vi "Ophir_calibration.vi"(10 "Адрес Ophir":refnum<visa-resource-name>="USB0::0x0BD3::0x0777::NI-VISA-10005::RAW", 11 "Путь к калибровке":path=path "D:/#mech/LVPROG/1991_Маэстро/Калибровка/Proj/Осциллограммы") -> ()   [LabVIEW 2013]
uses:
  <vilib>/Analysis/baseanly.llb/Mean (DBL).vi
  <vilib>/Utility/file.llb/Write To Spreadsheet File (DBL).vi
  <vilib>/Analysis/NI_AALBase.lvlib
panel:
  in  "X6 (N10)":dbl[][](array[numeric])=[[0.1, 2.0], [0.5, 2.0], [1.0, 2.0], [3.0, 2.0], [5.0, 2.0], [10.0, 2.0], [15.0, 2.0], [20.0, 2.0], [25.0, 2.0], [30.0, 2.0], [35.0, 2.0], [40.0, 2.0], [45.0, 20.0], [50.0, 20.0], [55.0, 20.0], [60.0, 20.0], [65.0, 20.0], [70.0, 20.0], [75.0, 20.0], [80.0, 20.0], [85.0, 20.0], [90.0, 20.0], [95.0, 20.0], [100.0, 20.0]] format="%0.3f"
  in  "Количество прострелов в импульсе":i32=40
  out "Минут":dbl=17.886183333333335
  in  "Boolean":bool=TRUE
  out "Предел":string="3"
  out "mean":dbl=2.91575 format="%0.2f"
  out "number 2":dbl=3.22e-06
  in  "number":i32
  out "Результат":string="*\n\n"
  in  "Телескоп":enum16{"X6", "X3", "X2", "X1"}(ring)
  in  "X1":dbl[][](array[numeric])=[[0.1, 20.0], [0.5, 200.0], [1.0, 200.0], [3.0, 2000.0], [5.0, 2000.0], [10.0, 2000.0], [15.0, 10000.0], [20.0, 10000.0], [25.0, 10000.0], [30.0, 10000.0], [35.0, 10000.0], [40.0, 10000.0], [45.0, 10000.0], [50.0, 10000.0], [55.0, 10000.0], [60.0, 10000.0], [65.0, 10000.0], [70.0, 10000.0], [75.0, 10000.0], [80.0, 10000.0], [85.0, 10000.0], [90.0, 10000.0], [95.0, 10000.0], [100.0, 10000.0]] format="%0.3f"
  in  "X2":dbl[][](array[numeric])=[[0.1, 20.0], [0.5, 200.0], [1.0, 200.0], [3.0, 200.0], [5.0, 2000.0], [10.0, 2000.0], [15.0, 2000.0], [20.0, 2000.0], [25.0, 2000.0], [30.0, 2000.0], [35.0, 2000.0], [40.0, 2000.0], [45.0, 10000.0], [50.0, 10000.0], [55.0, 10000.0], [60.0, 10000.0], [65.0, 10000.0], [70.0, 10000.0], [75.0, 10000.0], [80.0, 10000.0], [85.0, 10000.0], [90.0, 10000.0], [95.0, 10000.0], [100.0, 10000.0]] format="%0.3f"
  in  "X3":dbl[][](array[numeric])=[[0.1, 20.0], [0.5, 20.0], [1.0, 200.0], [3.0, 200.0], [5.0, 200.0], [10.0, 2000.0], [15.0, 2000.0], [20.0, 2000.0], [25.0, 2000.0], [30.0, 2000.0], [35.0, 2000.0], [40.0, 2000.0], [45.0, 2000.0], [50.0, 2000.0], [55.0, 2000.0], [60.0, 2000.0], [65.0, 2000.0], [70.0, 2000.0], [75.0, 2000.0], [80.0, 2000.0], [85.0, 2000.0], [90.0, 2000.0], [95.0, 2000.0], [100.0, 2000.0]] format="%0.3f"
  in  "X6":dbl[][](array[numeric])=[[0.1, 2.0], [0.5, 20.0], [1.0, 20.0], [3.0, 20.0], [5.0, 200.0], [10.0, 200.0], [15.0, 200.0], [20.0, 200.0], [25.0, 200.0], [30.0, 200.0], [35.0, 200.0], [40.0, 200.0], [45.0, 200.0], [50.0, 200.0], [55.0, 200.0], [60.0, 200.0], [65.0, 200.0], [70.0, 2000.0], [75.0, 2000.0], [80.0, 2000.0], [85.0, 2000.0], [90.0, 2000.0], [95.0, 2000.0], [100.0, 2000.0]] format="%0.3f"
  in  "USB Channel number (default 0)":dbl
  out "XY Graph":cluster{dbl[], dbl[]}(graph)={[45.0, 46.0, 47.0, 48.0, 49.0, 50.0, 51.0, 52.0, 53.0, 54.0, 55.0, 56.0, 57.0, 58.0, 59.0, 60.0, 61.0, 62.0, 63.0, 64.0, 65.0, 66.0, 67.0, 68.0, 69.0, 70.0, 71.0, 72.0, 73.0, 74.0, 75.0, 76.0, 77.0, 78.0, 79.0], [5.82625, 5.09275, 5.42575, 5.7905, 1.9792500000000002, 3.1294999999999997, 2.85025, 2.0719999999999996, 1.9745, 2.1955, 1.99275, 2.2165, 2.0700000000000003, 2.3114999999999997, 2.2840000000000003, 2.29225, 2.153, 2.2262500000000003, 2.49075, 2.4105, 2.2475, 2.3665000000000003, 2.592, 2.55425, 2.43575, 2.7362499999999996, 2.6025, 2.5602500000000004, 2.5745, 2.8725, 2.713, 2.661, 2.85275, 2.81675, 2.91575]}
  out "Текущий процент, %":dbl=79.0
  out "Шаг, %":dbl=1.0
  in  "Диапазон/Точки":bool=TRUE
  in  "Точки":dbl[](array[numeric])
  in  "Максимальный процент, %":dbl=80.0
  in  "Минимальный процент, %":dbl=45.0
  in  "Количество точек":u32=35
  in  "But_Автопрострел":bool=TRUE
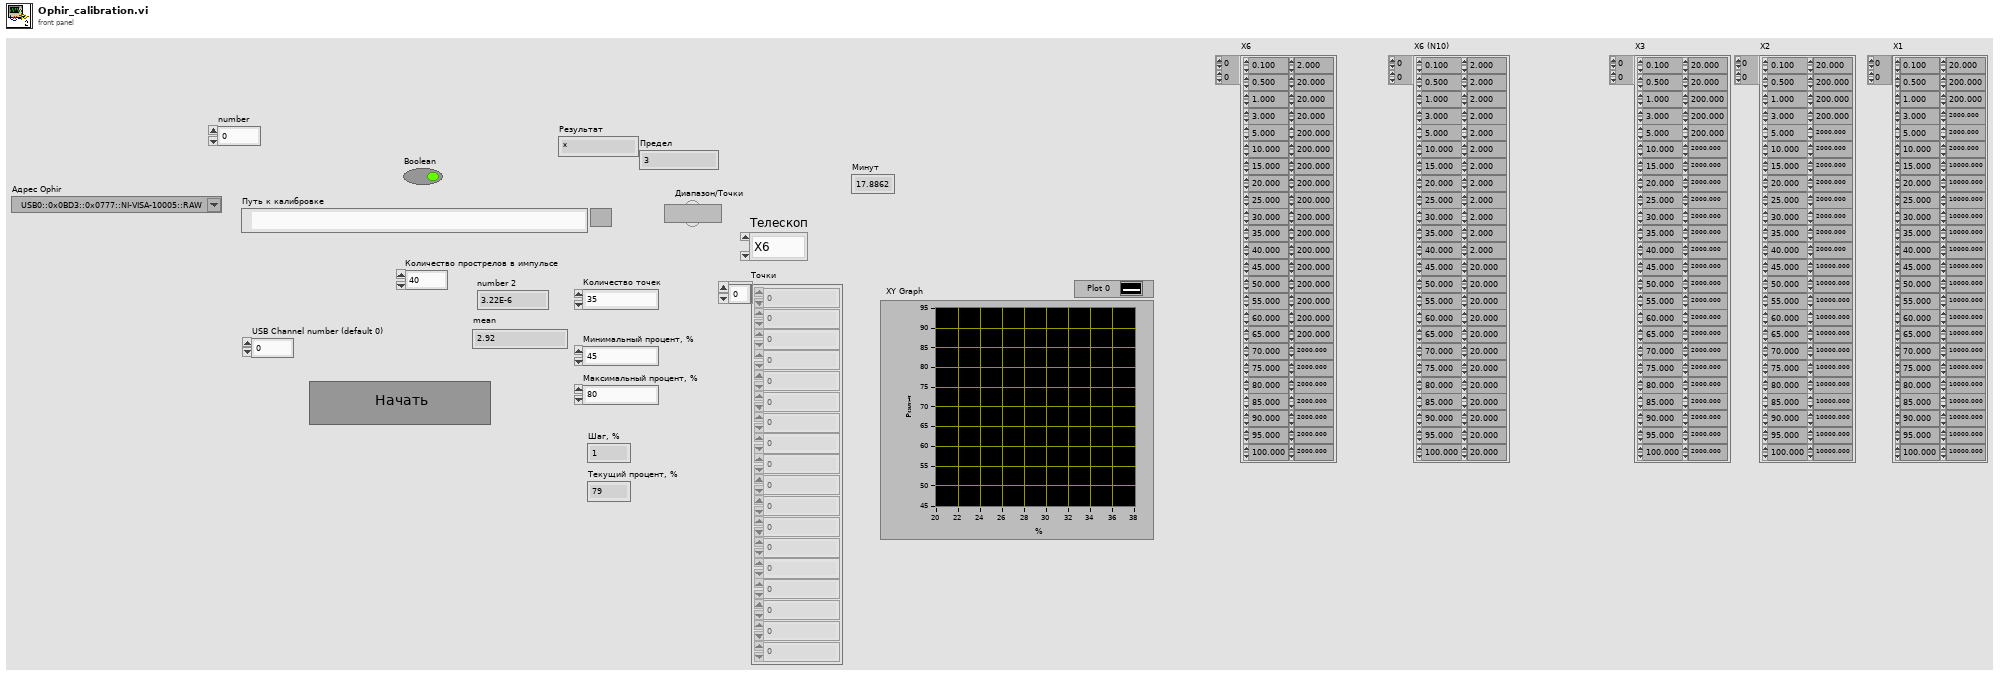
[diagram p1: front panel]
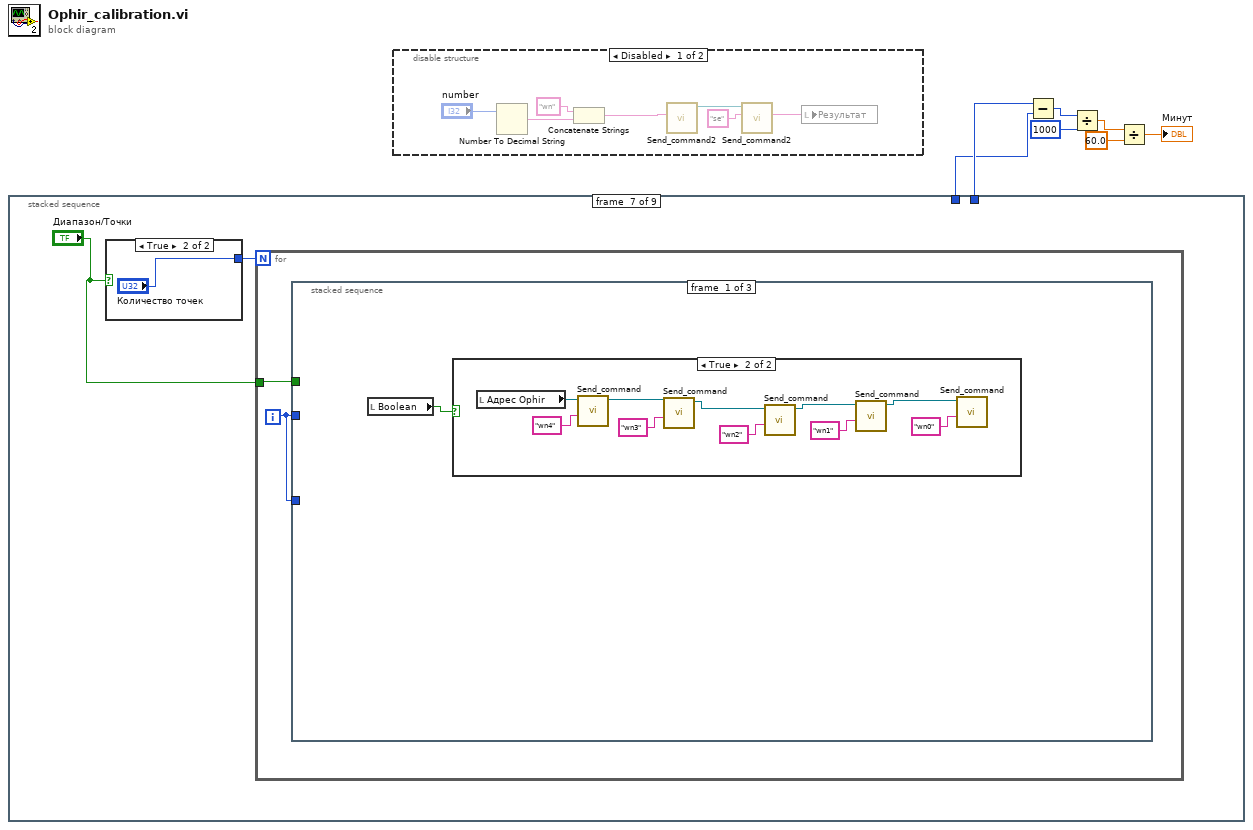
[diagram p0: block diagram]
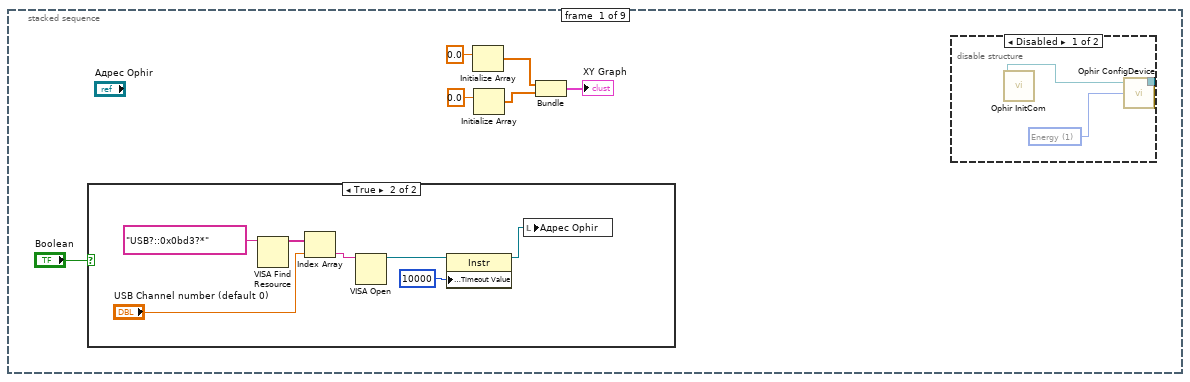
[diagram p3: hidden frame]
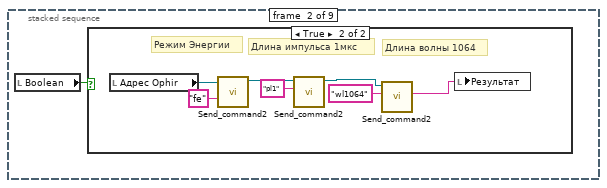
[diagram p6: hidden frame]
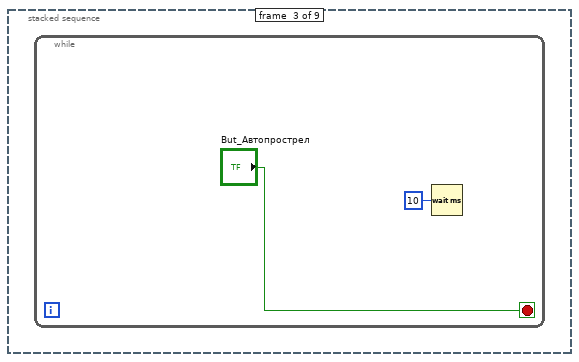
[diagram p8: hidden frame]
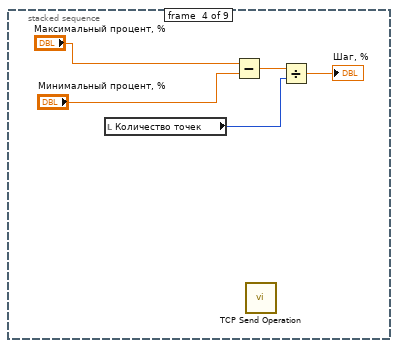
[diagram p9: hidden frame]
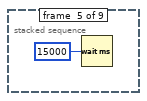
[diagram p10: hidden frame]
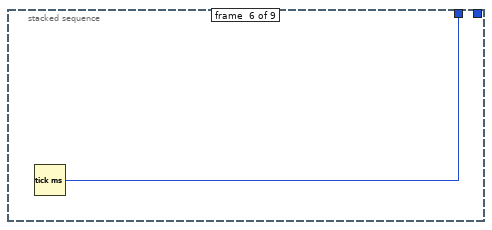
[diagram p11: hidden frame]
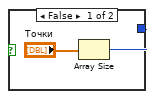
[diagram p12: hidden frame]
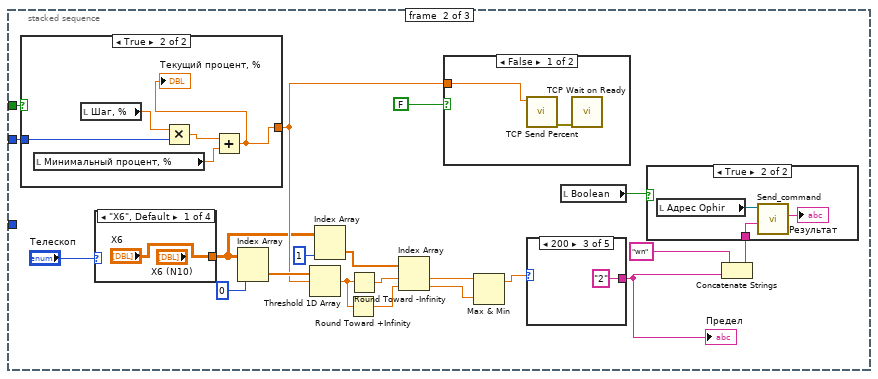
[diagram p14: hidden frame]
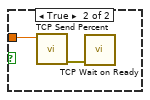
[diagram p16: hidden frame]
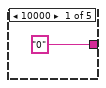
[diagram p17: hidden frame]
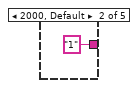
[diagram p18: hidden frame]
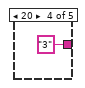
[diagram p19: hidden frame]
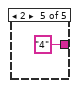
[diagram p20: hidden frame]
diagram:
  n1 = stacked-sequence {
    tunnel: [_ _ _ _ _ w40 _ _ _] -> w6
    tunnel: [_ _ _ _ _ _ _ w134 _] -> w7
    frame #0 {
      n2 = case shown="True" "Boolean" {
        frame False {
        }
        frame True {
          n3 = VISA Find Resource(11:"USB?::0x0bd3?*" ("USB0::0x0BD3")) -> (3:w16:string[])  [unwired: 1 in, 3 out]
          n4 = Index Array(array=w16, index="USB Channel number (default 0)") -> (element=w19:string)
          n5 = VISA Open(VISA resource name=w19) -> (VISA resource name=w20:refnum<visa-resource-name>)  [unwired: 1 in, 4 out]
          n6 = property class="Instr"(reference=w20, "General Settings:Timeout Value"=u32 10000) -> (reference out=w14:refnum<visa-resource-name>)  [unwired: 1 in, 1 out]
          n7 = local write "Адрес Ophir"(w14) -> ()
        }
      }
      n8 = Initialize Array(0.0 ("element")) -> (w11:dbl[])  [unwired: 1 in]
      n9 = Initialize Array(0.0 ("element")) -> (w10:dbl[])  [unwired: 1 in]
      n10 = Bundle(w11, w10) -> (→"XY Graph":cluster{dbl[], dbl[]})  [unwired: 1 in]
      n11 = disable-structure shown="Disabled" {
        disable-tunnel: [w21 _] -> _
        frame Disabled {
          w22 = u16 1 items=["Power", "Energy", "Frequency"] ("Measure Choice (0:Power)")
          n12 = call "Ophir InitCom.vi"() -> ("Visa Session"=w23:refnum<visa-resource-name>)  [unwired: 6 in, 2 out]
          n13 = call "Ophir ConfigDevice.vi"("Visa Session"=w23, "Measure Choice (0:Power)"=w22) -> ("dup Visa Session"=w21:refnum<visa-resource-name>)  [unwired: 1 in, 3 out]
        }
        frame Enabled {
        }
      }
    }
    frame #1 {
      n14 = local read "Boolean"() -> (w24:bool)
      n15 = case shown="True" w24 {
        frame False {
        }
        frame True {
          # "Длина волны 1064"
          # "Длина импульса 1мкс"
          # "Режим Энергии"
          n16 = local read "Адрес Ophir"() -> (w31:refnum<visa-resource-name>)
          n17 = call "Send_command2.vi"("String"="fe", "VISA Refnum in"=w31) -> ("VISA Refnum out"=w29:refnum<visa-resource-name>)  [unwired: 8 in, 1 out]
          n18 = call "Send_command2.vi"("String"="pl1", "VISA Refnum in"=w29) -> ("VISA Refnum out"=w26:refnum<visa-resource-name>)  [unwired: 8 in, 1 out]
          n19 = call "Send_command2.vi"("String"="wl1064", "VISA Refnum in"=w26) -> ("string"=w25:string)  [unwired: 8 in, 1 out]
          n20 = local write "Результат"(w25) -> ()
        }
      }
    }
    frame #2 {
      n21 = while {
        stop <- "But_Автопрострел" stop-if-true
        n22 = Wait (ms)(milliseconds to wait=u32 10) -> ()  [unwired: 1 out]
      }
    }
    frame #3 {
      n23 = local read "Количество точек"() -> (w37:u32)
      n24 = Subtract(x="Максимальный процент, %", y="Минимальный процент, %") -> (x-y=w36:dbl)
      n25 = call "TCP Send Operation.vi"() -> ()  [unwired: 11 in, 1 out]
      n26 = Divide(x=w36, y=w37) -> (x/y=→"Шаг, %":dbl)
    }
    frame #4 {
      n27 = Wait (ms)(milliseconds to wait=u32 15000) -> ()  [unwired: 1 out]
    }
    frame #5 {
      n28 = Tick Count (ms)() -> (millisecond timer value=w40:u32)
    }
    frame #6 {
      n29 = case shown="True" "Диапазон/Точки" {
        tunnel: [w43 "Количество точек"] -> w42
        frame False {
          n30 = Array Size(array="Точки") -> (size(s)=w43:i32)
        }
        frame True {
        }
      }
      n31 = for {
        N: w42 -> [_]
        tunnel: "Диапазон/Точки" -> [w47]
        i -> [w46]
        n32 = stacked-sequence {
          tunnel: w47 -> [_ w78 _]
          tunnel: w46 -> [_ w77 _]
          tunnel: w46 -> [_ _ w107]
          frame #0 {
            n33 = local read "Boolean"() -> (w48:bool)
            n34 = case shown="True" w48 {
              frame False {
              }
              frame True {
                n35 = local read "Адрес Ophir"() -> (w53:refnum<visa-resource-name>)
                n36 = call "Send_command.vi"("Команда"="wn4", "Адрес"=w53) -> ("Адрес 2"=w52:refnum<visa-resource-name>)  [unwired: 8 in, 1 out]
                n37 = call "Send_command.vi"("Команда"="wn3", "Адрес"=w52) -> ("Адрес 2"=w51:refnum<visa-resource-name>)  [unwired: 8 in, 1 out]
                n38 = call "Send_command.vi"("Команда"="wn2", "Адрес"=w51) -> ("Адрес 2"=w50:refnum<visa-resource-name>)  [unwired: 8 in, 1 out]
                n39 = call "Send_command.vi"("Команда"="wn1", "Адрес"=w50) -> ("Адрес 2"=w49:refnum<visa-resource-name>)  [unwired: 8 in, 1 out]
                n40 = call "Send_command.vi"("Команда"="wn0", "Адрес"=w49) -> ()  [unwired: 8 in, 2 out]
              }
            }
          }
          frame #1 {
            n41 = case shown="True" w78 {
              tunnel: w77 -> [w96 w100]
              tunnel: [w95 w98] -> w73
              frame False {
                n42 = local read "Точки"() -> (w97:dbl[])
                n43 = Index Array(array=w97, index=w96) -> (element=w95:dbl)
              }
              frame True {
                n44 = local read "Минимальный процент, %"() -> (w102:dbl)
                n45 = local read "Шаг, %"() -> (w101:dbl)
                n46 = Multiply(x=w101, y=w100) -> (x*y=w99:dbl)
                n47 = Add(x=w99, y=w102) -> (x+y=w98:dbl)
                "Текущий процент, %" <- w98
              }
            }
            n48 = case shown="\"X6\", Default" "Телескоп" {
              tunnel: ["X6" "X3" "X2" "X1"] -> w72
              frame "X6", Default {
              }
              frame "X3" {
              }
              frame "X2" {
              }
              frame "X1" {
              }
            }
            n49 = Index Array(array=w72, index (col)=0 ("disabled index (col)")) -> (element=w74:dbl[])  [unwired: 1 in]
            n50 = Threshold 1D Array(2:w73, 3:w74) -> (0:w68:dbl)  [unwired: 1 in]
            n51 = Index Array(array=w72, index (col)=1 ("disabled index (col)")) -> (element=w70:dbl[])  [unwired: 1 in]
            n52 = Round Toward +Infinity(x=w68) -> (ceil(x): smallest int >= x=w67:dbl)
            n53 = Round Toward -Infinity(1:w68) -> (0:w69:dbl)
            n54 = Index Array(array=w70, index #1=w69, index #2=w67) -> (element #1=w66:dbl, element #2=w65:dbl)
            n55 = case shown="False" FALSE {
              tunnel: w73 -> [w83 w84]
              frame False {
                n56 = call "TCP Send Percent.vi"("Percent"=w83) -> ("error out"=w82:errorcluster)  [unwired: 10 in]
                n57 = call "TCP Wait on Ready.vi"("error in"=w82) -> ()  [unwired: 9 in, 1 out]
              }
              frame True {
                n58 = call "TCP Send Percent.vi"("Percent"=w84) -> ("error out"=w85:errorcluster)  [unwired: 10 in]
                n59 = call "TCP Wait on Ready.vi"("error in"=w85) -> ()  [unwired: 9 in, 1 out]
              }
            }
            n60 = Max & Min(x=w66, y=w65) -> (max(x,y)=w64:dbl)  [unwired: 1 out]
            n61 = case shown="200" w64 {
              tunnel: ["0" "1" "2" "3" "4"] -> w62
              frame 10000 {
              }
              frame 2000, Default {
              }
              frame 200 {
              }
              frame 20 {
              }
              frame 2 {
              }
            }
            "Предел" <- w62
            n62 = local read "Boolean"() -> (w59:bool)
            n63 = Concatenate Strings("wn", w62) -> (w61:string)
            n64 = case shown="True" w59 {
              tunnel: w61 -> [_ w81]
              frame False {
              }
              frame True {
                n65 = local read "Адрес Ophir"() -> (w80:refnum<visa-resource-name>)
                n66 = call "Send_command.vi"("Команда"=w81, "Адрес"=w80) -> ("Результат"=→"Результат":string)  [unwired: 8 in, 1 out]
              }
            }
          }
          frame #2 {
            n67 = local read "Boolean"() -> (w103:bool)
            n68 = for {
              N: "Количество прострелов в импульсе" -> [_]
              tunnel: [w118] -> w115 mode=indexing
              tunnel: w103 -> [w117]
              n69 = stacked-sequence {
                tunnel: [_ _ _ w126] -> w118
                tunnel: w117 -> [w119 _ _ _]
                tunnel: w117 -> [_ _ _ w125]
                frame #0 {
                  n70 = case shown="True" w119 {
                    frame False {
                    }
                    frame True {
                      n71 = local read "Предел"() -> (w120:string)
                      n72 = local read "Адрес Ophir"() -> (w122:refnum<visa-resource-name>)
                      n73 = Concatenate Strings("wn", w120) -> (w121:string)
                      n74 = call "Send_command.vi"("Команда"=w121, "Адрес"=w122) -> ()  [unwired: 8 in, 2 out]
                    }
                  }
                }
                frame #1 {
                  n75 = call "TCP Send Fire.vi"() -> ()  [unwired: 11 in, 1 out]
                }
                frame #2 {
                  n76 = Wait (ms)(milliseconds to wait=u32 300) -> ()  [unwired: 1 out]
                }
                frame #3 {
                  n77 = case shown="False" w125 {
                    tunnel: ["" ("string") w133] -> w127
                    frame False {
                    }
                    frame True {
                      n78 = local read "Адрес Ophir"() -> (w131:refnum<visa-resource-name>)
                      n79 = call "Send_command2.vi"("String"="se" ("string"), "VISA Refnum in"=w131) -> ("string"=w133:string)  [unwired: 8 in, 1 out]
                    }
                  }
                  n80 = Fract/Exp String To Number(use system decimal point (T)=FALSE, string=w127, offset=1) -> (number=w126:dbl)  [unwired: 2 out]
                  "number 2" <- w126
                }
              }
            }
            n81 = local read "Текущий процент, %"() -> (w112:dbl)
            n82 = call-poly <vilib>:"Mean.vi"("X"=w115) -> ("mean"=w106:dbl)  [unwired: 1 out]
            n83 = Multiply(x=w106, y=1000000.0) -> (x*y=w104:dbl)
            "mean" <- w104
            n84 = local read "XY Graph"() -> (w114:cluster{dbl[], dbl[]})
            n85 = Unbundle(w114) -> (w113:dbl[], w111:dbl[])
            n86 = Insert Into Array(array=w113, index=w107, new element=w112) -> (w110:dbl[])
            n87 = Insert Into Array(array=w111, index=w107, new element=w104) -> (w109:dbl[])
            n88 = Bundle(w110, w109) -> (w108:cluster{dbl[], dbl[]})  [unwired: 1 in]
            n89 = local write "XY Graph"(w108) -> ()
          }
        }
      }
    }
    frame #7 {
      n90 = Tick Count (ms)() -> (millisecond timer value=w134:u32)
    }
    frame #8 {
      n91 = call <vilib>:"Check if File or Folder Exists.vi"("path"="Путь к калибровке") -> ("file or folder exists?"=w143:bool, "dup path"=w142:path)  [unwired: 8 in, 1 out]
      n92 = Get Date/Time In Seconds() -> (seconds since 1Jan1904=w154:timestamp)
      n93 = case shown="False" w143 {
        tunnel: w142 -> [w156 w157]
        tunnel: [w155 w157] -> w141
        frame False {
          n94 = Create Folder(path (use dialog)=w156) -> (created path=w155:path)  [unwired: 2 in, 2 out]
        }
        frame True {
        }
      }
      n95 = Format Date/Time String(time format string (%c)="%d_%m_%y  %H;%M;%S", seconds (now)=w154) -> (date/time string=w152:string)  [unwired: 1 in]
      n96 = Concatenate Strings("Калибровка" ("string"), "_" ("string"), w152, ".xls" ("string")) -> (w149:string)
      n97 = local read "XY Graph"() -> (w148:cluster{dbl[], dbl[]})
      n98 = Build Path(base path=w141, name or relative path=w149) -> (appended path=w136:path)
      n99 = Unbundle(w148) -> (w147:dbl[], w146:dbl[])
      n100 = Build Array(w147, w146) -> (w138:dbl[][])
      n101 = call-poly <vilib>:"Write To Spreadsheet File.vi"("transpose? (no:F)"=TRUE, "format (%.3f)"="%.9f", "2D data"=w138, "file path (dialog if empty)"=path "D:/#mech/LVPROG/1991_Маэстро/Калибровка/Осциллограммы/5.xls") -> ()  [unwired: 4 in, 1 out]
      n102 = call-poly <vilib>:"Write To Spreadsheet File.vi"("transpose? (no:F)"=TRUE, "2D data"=w138, "file path (dialog if empty)"=w136) -> ()  [unwired: 5 in, 1 out]
    }
  }
  n103 = disable-structure shown="Disabled" {
    frame Disabled {
      n104 = Number To Decimal String(number="number") -> (decimal integer string=w158:string)  [unwired: 1 out]
      n105 = Concatenate Strings("wn", w158) -> (w160:string)
      n106 = call "Send_command2.vi"("String"=w160) -> ("VISA Refnum out"=w162:refnum<visa-resource-name>)  [unwired: 9 in, 1 out]
      n107 = call "Send_command2.vi"("String"="se" ("string"), "VISA Refnum in"=w162) -> ("string"=w164:string)  [unwired: 8 in, 1 out]
      n108 = local write "Результат"(w164) -> ()
    }
    frame Enabled {
    }
  }
  n109 = Subtract(x=w7, y=w6) -> (x-y=w5:u32)
  n110 = Divide(x=w5, y=u32 1000) -> (x/y=w3:dbl)
  n111 = Divide(x=w3, y=60.0) -> (x/y=→"Минут":dbl)
